vi "Get Query (datea range).vi"(9 "End time":timestamp format="%<%.3X\n%y/%m/%d>T", 11 "Start time":timestamp format="%<%.3X\n%y/%m/%d>T") -> (2 "Qwery":string)   [LabVIEW 2017]
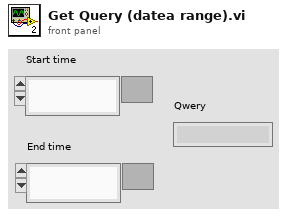
[diagram p1: front panel]
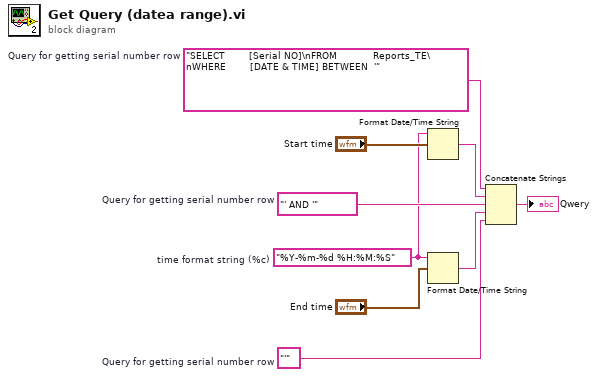
[diagram p0: block diagram]
diagram:
  w4 = "%Y-%m-%d %H:%M:%S"  # time format string (%c)
  w9 = "'"  # Query for getting serial number row
  w8 = "' AND '"  # Query for getting serial number row
  w7 = "SELECT        [Serial NO]\nFROM            Reports_TE\nWHERE        [DATE & TIME] BETWEEN  '"  # Query for getting serial number row
  n1 = Format Date/Time String(time format string (%c)=w4, seconds (now)="Start time") -> (date/time string=w3:string)  [unwired: 1 in]
  n2 = Format Date/Time String(time format string (%c)=w4, seconds (now)="End time") -> (date/time string=w2:string)  [unwired: 1 in]
  n3 = Concatenate Strings(w7, w3, w8, w2, w9) -> (→"Qwery":string)
